vi "serial_init.vi"(7 "clear?":bool, 8 "VISA resource name":refnum<visa-resource-name>="COM7") -> (0 "VISA resource name out":refnum<visa-resource-name>)   [LabVIEW 2021]
uses:
  <vilib>/Instr/_visa.llb/VISA Configure Serial Port (Instr).vi
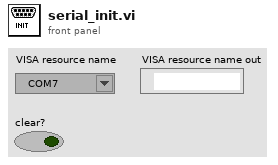
[diagram p1: front panel]
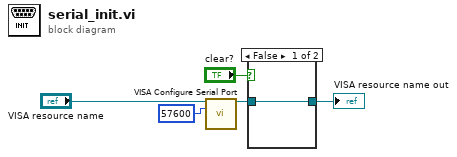
[diagram p0: block diagram]
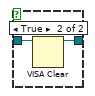
[diagram p2: hidden frame]
diagram:
  n1 = call-poly "VISA Configure Serial Port"("VISA resource name"="VISA resource name", "baud rate (9600)"=u32 57600) -> ("VISA resource name out"=w3:refnum<visa-resource-name>)  [unwired: 12 in, 1 out]
  n2 = case shown="False" "clear?" {
    tunnel: w3 -> [w6 w8]
    tunnel: [w6 w7] -> w1
    frame False {
    }
    frame True {
      n3 = VISA Clear(VISA resource name=w8) -> (VISA resource name out=w7:refnum<visa-resource-name>)  [unwired: 1 in, 1 out]
    }
  }
  "VISA resource name out" <- w1
